vi "testp2p.vi"() -> ()   [LabVIEW 2018]
uses:
  AdvSessionResources/AdvSessionResources/Adv Session Resources/14.0/english/labview2014/win32U/Nodes/ResourceInfo.ctl
  AdvSessionResources/AdvSessionResources/Adv Session Resources/14.0/english/labview2014/win32U/Nodes/OpenByNameSubVI.vi
  AdvSessionResources/AdvSessionResources/Adv Session Resources/14.0/english/labview2014/win32U/Nodes/OpenByName.xnode
  AdvSessionResources/AdvSessionResources/Adv Session Resources/14.0/english/labview2014/win32U/Nodes/LVFPGAAdvSessionResources.lvlib
panel:
  out "Error out":errorcluster
  in  "fifo":string="p2p writer"
  in  "File Path":path=path "C:/Program Files (x86)/National Instruments/LabVIEW 2018/examples/R Series/Device Specific/PXIe MIO Devices/Peer to Peer Loopback/FPGA Bitfiles/FPGAWriter.lvbitx"
  in  "Device address":string="7820_2"
  out "Registers found":string[](array[string])=["Data", "Samples Sent", "Element", "p2p writer"]
  out "Resource info out":T1[](array[typedef])=[{"Resource name"="Data", "Data type"=variant(fxp<+/-,27,5> 0.0), "Resource type"=enum."Register"}, {"Resource name"="Samples Sent", "Data type"=variant(u64 0), "Resource type"=enum."Register"}, {"Resource name"="Element", "Data type"=variant(fxp<+/-,27,5> 0.0), "Resource type"=enum."Register"}, {"Resource name"="p2p writer", "Data type"=variant(fxp<+/-,27,5> 0.0), "Resource type"=enum."Host To Target FIFO"}]
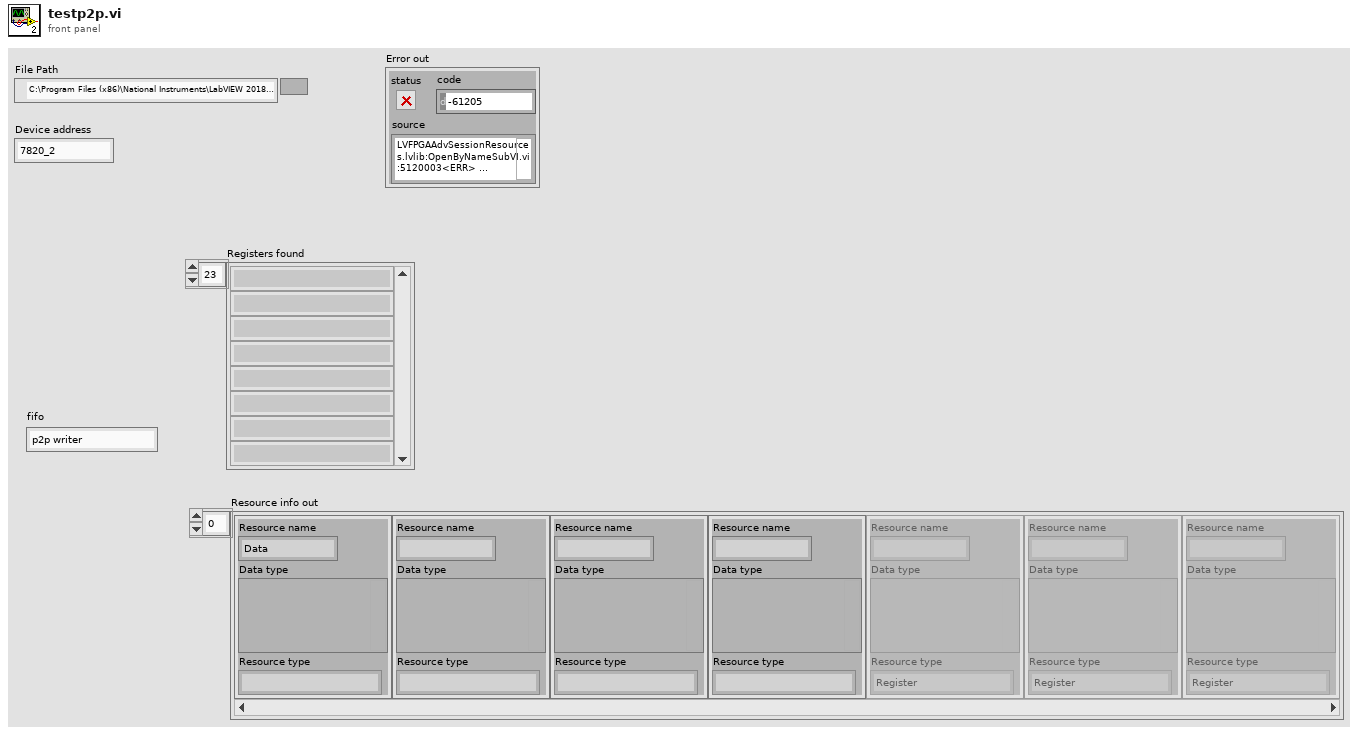
[diagram p1: front panel]
types:
  T1 = typedef "LVFPGAAdvSessionResources.lvlib/ResourceInfo.ctl" = cluster{"Resource name":string, "Data type":variant, "Resource type":enum16{"Register", "Host To Target FIFO", "Target To Host FIFO"}}
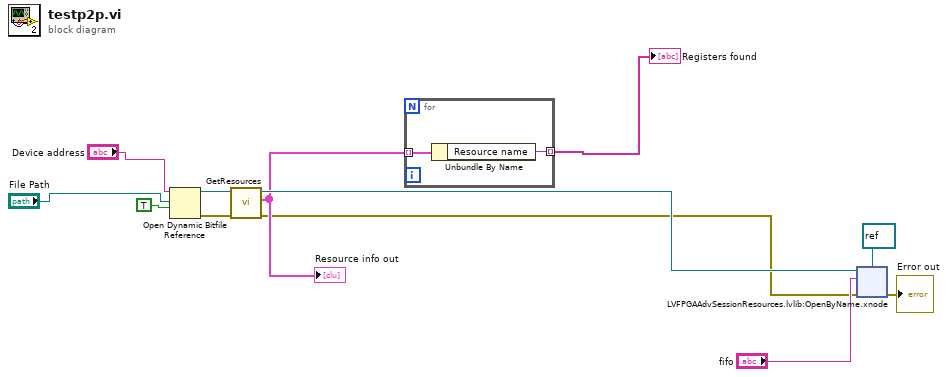
[diagram p0: block diagram]
diagram:
  n1 = Open Dynamic Bitfile Reference(0:"Device address", 1:"File Path", 2:TRUE ("Run When Loaded")) -> (5:w10:refnum<k20>, 8:w11:errorcluster)  [unwired: 2 in]
  n2 = call "GetResources.vi"("error in (no error)"=w11, "FPGA VI Reference in"=w10) -> ("error out"=w1:errorcluster, "Resource info out"=w3:T1[], "FPGA VI Reference out"=w4:refnum<k20>)  [unwired: 7 in]
  "Resource info out" <- w3
  n3 = for {
    tunnel: w3 -> [w14] mode=indexing
    tunnel: [w13] -> w9 mode=indexing
    n4 = Unbundle By Name(w14) -> ("Resource name"=w13:string)
  }
  "Registers found" <- w9
  n5 = xnode "LVFPGAAdvSessionResources.lvlib:OpenByName.xnode"("FPGA VI Reference in"=w4, "Resource name in"="fifo", "Single resource reference type in"=refnum<k20> refnum, "Error in"=w1) -> ("Error out"=→"Error out":errorcluster)  [unwired: 2 out]
